vi "dfd_SOS to ZPK.vi"(10 "reverse coefficients":dbl[](array[numeric]) format="%.2f", 11 "forward coefficients":dbl[](array[numeric]) format="%.2f") -> (1 "k":dbl format="%.2f", 2 "poles":cdb[](array[numeric]) format="%.2f", 3 "zeros":cdb[](array[numeric]) format="%.2f")   [LabVIEW 2017, in "NI_DigFilterLicensed.lvlib"]
uses:
  <vilib>/addons/Digital Filter Design/NI_DigFilterLicensed.lvlib
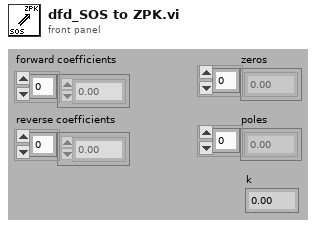
[diagram p1: front panel]
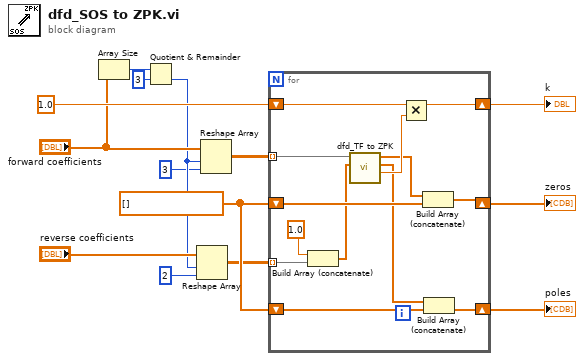
[diagram p0: block diagram]
diagram:
  w10 = cdb[] []
  n1 = Array Size(array="forward coefficients") -> (size(s)=w12:i32)
  n2 = Quotient & Remainder(x=w12, y=3) -> (floor(x/y)=w3:i32)  [unwired: 1 out]
  n3 = Reshape Array("reverse coefficients", w3, 2 ("dimension size")) -> (w4:dbl[][])
  n4 = Reshape Array("forward coefficients", w3, 3 ("dimension size")) -> (w6:dbl[][])
  n5 = for {
    shift-right: [w26] -> w9
    shift-left: w10 -> [w27]
    shift-right: [w24] -> w8
    shift-left: w10 -> [w25]
    tunnel: w4 -> [w15] mode=indexing
    shift-right: [w22] -> w13
    shift-left: 1.0 ("gain") -> [w23]
    tunnel: w6 -> [w16] mode=indexing
    n6 = Build Array (concatenate)(1.0, w15) -> (w17:dbl[])
    n7 = call <vilib>:"dfd_TF to ZPK.vi"("denominator"=w17, "numerator"=w16) -> ("gain"=w21:dbl, "poles"=w19:cdb[], "zeros"=w20:cdb[])  [unwired: 7 out]
    n8 = Multiply(x=w23, y=w21) -> (x*y=w22:dbl)
    n9 = Build Array (concatenate)(w20, w27) -> (w26:cdb[])
    n10 = Build Array (concatenate)(w19, w25) -> (w24:cdb[])
  }
  "poles" <- w8
  "zeros" <- w9
  "k" <- w13
